vi "HeadingSubVI.vi"(8 "error in (no error)":errorcluster, 11 "PmodCMPS address":u8) -> (0 "error out":errorcluster, 1 "Heading Shifted":dbl, 2 "Heading Stretched":dbl, 3 "Heading Raw":dbl, 5 "Blimp Orientation":dbl)   [LabVIEW 2015]
uses:
  <vilib>/myRIO/Instrument Drivers/Onboard IO/DIO/vis/Read.vi
  <vilib>/myRIO/Instrument Drivers/Onboard IO/I2C/vis/Configure.vi
  <vilib>/myRIO/Instrument Drivers/Onboard IO/I2C/vis/Write Read.vi
  <vilib>/myRIO/Instrument Drivers/Onboard IO/DIO/vis/Smart Open.vi
  <vilib>/Utility/error.llb/Error Cluster From Error Code.vi
  <vilib>/myRIO/Common/Instrument Driver Framework/myRIO v1.0/DIO/vis/myRIO v1.0 Read DIO.vi
  <vilib>/myRIO/Instrument Drivers/Onboard IO/I2C/vis/Smart Open.vi
  <vilib>/myRIO/Common/Instrument Driver Framework/myRIO v1.0/I2C/vis/myRIO v1.0 Configure I2C.vi
  <vilib>/myRIO/Common/Instrument Driver Framework/myRIO v1.0/I2C/vis/myRIO v1.0 Write I2C.vi
  <vilib>/myRIO/Common/Instrument Driver Framework/myRIO v1.0/I2C/vis/myRIO v1.0 Read I2C.vi
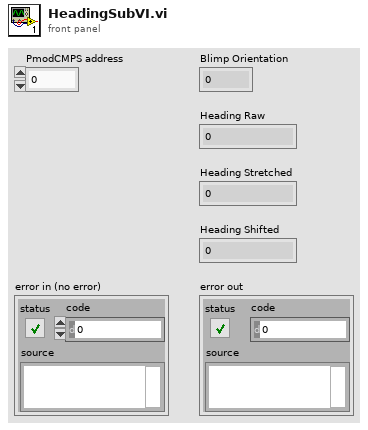
[diagram p1: front panel]
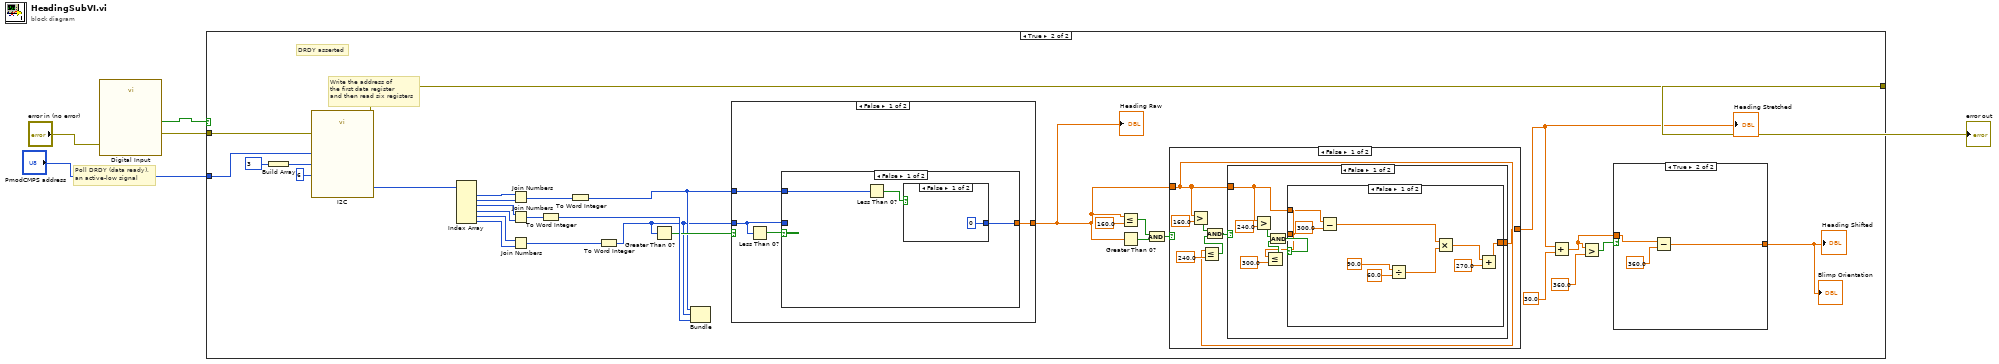
[diagram p0: block diagram]
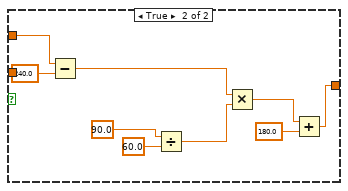
[diagram p4: hidden frame]
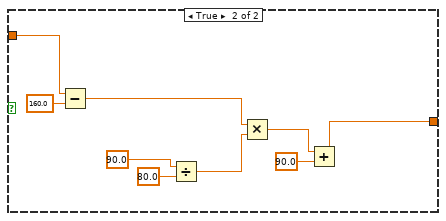
[diagram p5: hidden frame]
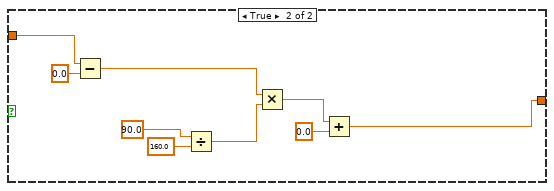
[diagram p6: hidden frame]
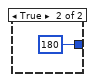
[diagram p7: hidden frame]
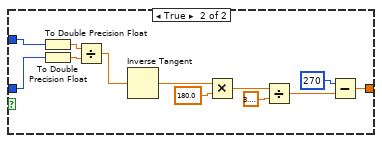
[diagram p8: hidden frame]
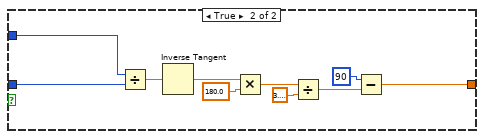
[diagram p9: hidden frame]
diagram:
  # "Poll DRDY (data ready),\nan active-low signal"
  n1 = call "Digital Input"("error in (no error)"="error in (no error)") -> ("A/DIO0 (Pin 11)"=w5:bool, "error out"=w4:errorcluster)  [unwired: 25 in]
  n2 = case shown="True" w5 {
    tunnel: "PmodCMPS address" -> [_ w37]
    tunnel: w4 -> [w6 w26]
    tunnel: [w6 w22] -> w3
    frame False {
      # "DRDY deasserted"
    }
    frame True {
      # "DRDY asserted"
      # "Write the address of\nthe first data register\nand then read six registers"
      n3 = Build Array(u8 3) -> (w23:u8[])
      n4 = call "I2C"("Slave Address (7-bit)"=w37, "Bytes to Write"=w23, "Byte Count"=u32 6, "error in (no error)"=w26) -> ("Bytes Read"=w27:u8[], "error out"=w22:errorcluster)  [unwired: 22 in]
      n5 = Index Array "Index Array"(array=w27) -> (element #1=w36:u8, element #2=w35:u8, element #3=w33:u8, element #4=w32:u8, element #5=w31:u8, element #6=w30:u8)  [unwired: 6 in]
      n6 = Join Numbers(hi=w36, lo=w35) -> ((hi.lo)=w34:u16)
      n7 = Join Numbers(hi=w33, lo=w32) -> ((hi.lo)=w29:u16)
      n8 = Join Numbers(hi=w31, lo=w30) -> ((hi.lo)=w28:u16)
      n9 = To Word Integer(number=w29) -> (16bit integer=w21:i16)
      n10 = To Word Integer(number=w34) -> (16bit integer=w19:i16)
      n11 = To Word Integer(number=w28) -> (16bit integer=w18:i16)
      n12 = Greater Than 0?(x=w18) -> (x > 0?=w20:bool)
      n13 = Bundle(w19, w18, w21) -> ()  [unwired: 1 in, 1 out]
      n14 = case shown="False" w20 {
        tunnel: w19 -> [w93 w115]
        tunnel: w18 -> [w92 w114]
        tunnel: [w94 w113] -> w13
        frame False {
          n15 = Less Than 0?(x=w92) -> (x < 0?=w95:bool)
          n16 = case shown="False" w95 {
            tunnel: [w96 w105] -> w94
            tunnel: w93 -> [w98 w104]
            tunnel: w92 -> [_ w102]
            frame False {
              n17 = Less Than 0?(x=w98) -> (x < 0?=w97:bool)
              n18 = case shown="False" w97 {
                tunnel: [0 180] -> w96
                frame False {
                }
                frame True {
                }
              }
            }
            frame True {
              n19 = To Double Precision Float(number=w104) -> (double precision float=w103:dbl)
              n20 = To Double Precision Float(number=w102) -> (double precision float=w101:dbl)
              n21 = Divide(x=w103, y=w101) -> (x/y=w106:dbl)
              n22 = Inverse Tangent(1:w106) -> (0:w107:dbl)
              n23 = Multiply(x=w107, y=180.0) -> (x*y=w110:dbl)
              n24 = Divide(x=w110, y=3.141592653589793) -> (x/y=w108:dbl)
              n25 = Subtract(x=270, y=w108) -> (x-y=w105:dbl)
            }
          }
        }
        frame True {
          n26 = Divide(x=w115, y=w114) -> (x/y=w116:dbl)
          n27 = Inverse Tangent(1:w116) -> (0:w117:dbl)
          n28 = Multiply(x=w117, y=180.0) -> (x*y=w120:dbl)
          n29 = Divide(x=w120, y=3.141592653589793) -> (x/y=w118:dbl)
          n30 = Subtract(x=90, y=w118) -> (x-y=w113:dbl)
        }
      }
      "Heading Raw" <- w13
      n31 = Less Or Equal?(x=w13, y=160.0) -> (x <= y?=w16:bool)
      n32 = Greater Than 0?(x=w13) -> (x > 0?=w17:bool)
      n33 = And(x=w16, y=w17) -> (x .and. y?=w14:bool)
      n34 = case shown="False" w14 {
        tunnel: w13 -> [w43 w90]
        tunnel: [w42 w83] -> w12
        frame False {
          n35 = Greater?(x=w43, y=160.0) -> (0:w47:bool)
          n36 = Less Or Equal?(x=w43, y=240.0) -> (x <= y?=w44:bool)
          n37 = And(x=w47, y=w44) -> (x .and. y?=w48:bool)
          n38 = case shown="False" w48 {
            tunnel: w43 -> [w49 w74]
            tunnel: [w50 w75] -> w42
            frame False {
              n39 = Greater?(x=w49, y=240.0) -> (0:w55:bool)
              n40 = Less Or Equal?(x=w49, y=300.0) -> (x <= y?=w51:bool)
              n41 = And(x=w55, y=w51) -> (x .and. y?=w52:bool)
              n42 = case shown="False" w52 {
                tunnel: [w56 w65] -> w50
                tunnel: w49 -> [_ _]
                tunnel: w49 -> [w57 w66]
                frame False {
                  n43 = Subtract(x=w57, y=300.0) -> (x-y=w61:dbl)
                  n44 = Divide(x=90.0 ("y"), y=60.0) -> (x/y=w60:dbl)
                  n45 = Multiply(x=w61, y=w60) -> (x*y=w59:dbl)
                  n46 = Add(x=w59, y=270.0) -> (x+y=w56:dbl)
                }
                frame True {
                  n47 = Subtract(x=w66, y=240.0) -> (x-y=w70:dbl)
                  n48 = Divide(x=90.0 ("y"), y=60.0) -> (x/y=w69:dbl)
                  n49 = Multiply(x=w70, y=w69) -> (x*y=w68:dbl)
                  n50 = Add(x=w68, y=180.0) -> (x+y=w65:dbl)
                }
              }
            }
            frame True {
              n51 = Subtract(x=w74, y=160.0) -> (x-y=w79:dbl)
              n52 = Divide(x=90.0 ("y"), y=80.0) -> (x/y=w78:dbl)
              n53 = Multiply(x=w79, y=w78) -> (x*y=w77:dbl)
              n54 = Add(x=w77, y=90.0) -> (x+y=w75:dbl)
            }
          }
        }
        frame True {
          n55 = Subtract(x=w90, y=0.0) -> (x-y=w87:dbl)
          n56 = Divide(x=90.0 ("y"), y=160.0) -> (x/y=w86:dbl)
          n57 = Multiply(x=w87, y=w86) -> (x*y=w85:dbl)
          n58 = Add(x=w85, y=0.0) -> (x+y=w83:dbl)
        }
      }
      "Heading Stretched" <- w12
      n59 = Add(x=w12, y=30.0) -> (x+y=w11:dbl)
      n60 = Greater?(x=w11, y=360.0) -> (0:w9:bool)
      n61 = case shown="True" w9 {
        tunnel: w11 -> [w38 w41]
        tunnel: [w38 w39] -> w7
        frame False {
        }
        frame True {
          n62 = Subtract(x=w41, y=360.0) -> (x-y=w39:dbl)
        }
      }
      "Heading Shifted" <- w7
      "Blimp Orientation" <- w7
    }
  }
  "error out" <- w3
